vi "Analyzer.TestLauncher.vi"() -> ()   [LabVIEW 2022 SP3, in "Analyzer.lvclass"]
uses:
  Analyzer.lvclass
  Typedefs/Analyzer State--enum.ctl
  <vilib>/JKI/JKI SMO/SMO/Typedefs/SMOState --Enum.ctl
  C:/Program Files (x86)/National Instruments/LabVIEW 2022/vi.lib/JKI/JKI SMO/SMO/SMO.lvclass
  <vilib>/JKI/JKI SMO/SMO/SMO.lvclass/SMO.ctl
  <vilib>/JKI/JKI SMO/SMO/Private/ReftoDVR--SMO.vi
  Analyzer.lvclass/Analyzer.ctl
  <vilib>/JKI/JKI SMO/SMO/SMO.lvclass
panel:
  out "Time":dbl
  out "SMO State":T1
  in  "Embed?":bool=TRUE
  out "UI State":T2
  out "error out":errorcluster
  in  "Stop":bool
  # "SMO.UI_Embedded Test Launcher"
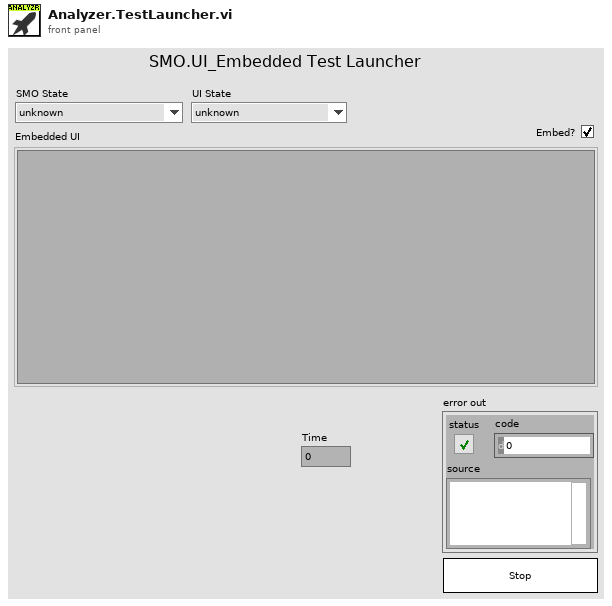
[diagram p1: front panel]
types:
  T1 = typedef "SMO.lvclass/SMOState --Enum.ctl" = enum16{"unknown", "Created", "Started", "Stopped"}
  T2 = typedef "Analyzer.lvclass/Analyzer State--enum.ctl" = enum16{"unknown", "Opened", "Embedded", "Closed"}
  T3 = typedef "SMO.lvclass/Public Events.ctl" = cluster{"Error":refnum<user-event>, "State":refnum<user-event>, "Reserve State":refnum<user-event>}
  T4 = typedef "Analyzer.lvclass/PublicEvents--Cluster.ctl" = cluster{"UI State":refnum<user-event>, "NewEventMessage":refnum<user-event>}
  T5 = cluster{"Event Registration Refnum":refnum<event-registration>}
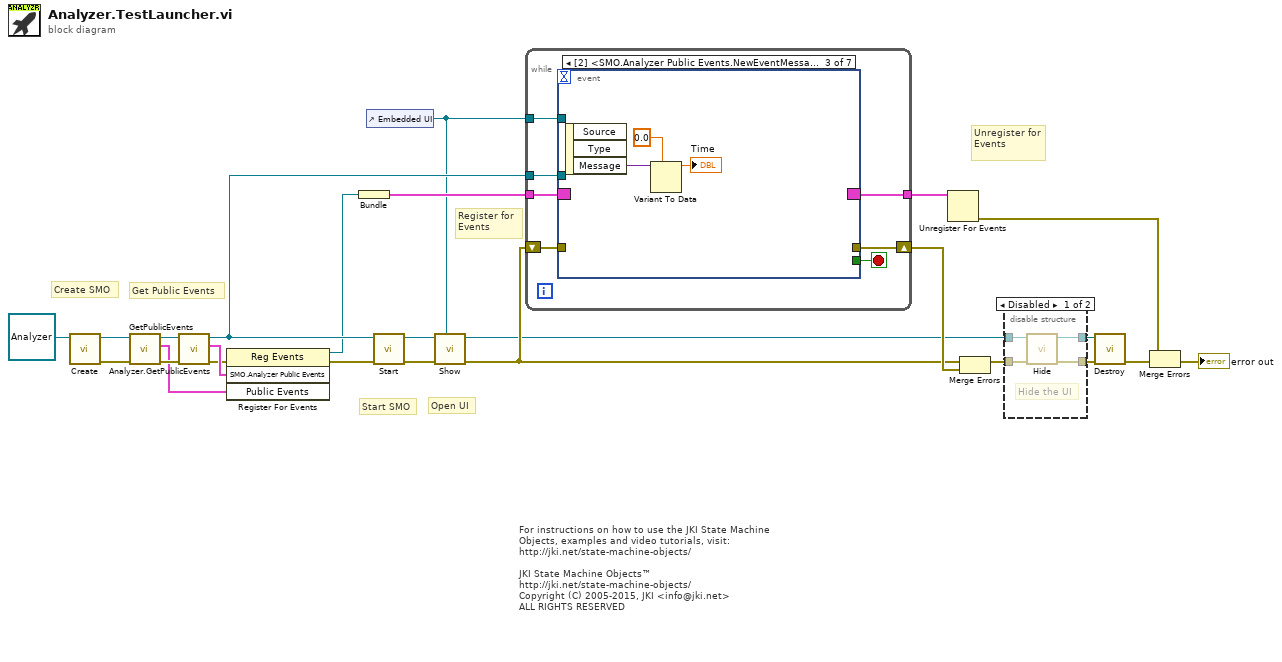
[diagram p0: block diagram]
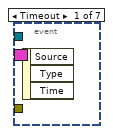
[diagram p3: hidden frame]
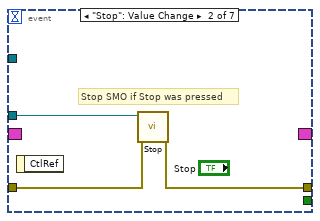
[diagram p4: hidden frame]
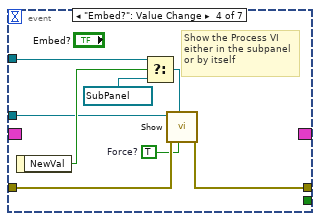
[diagram p5: hidden frame]
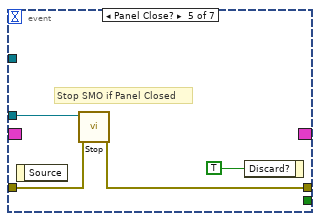
[diagram p6: hidden frame]
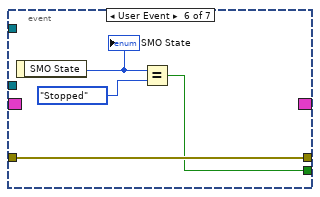
[diagram p7: hidden frame]
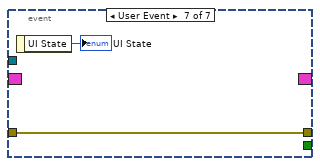
[diagram p8: hidden frame]
diagram:
  # "For instructions on how to use the JKI State Machine Objects, examples and video tutorials, visit:\nhttp://jki.net/state-machine-objects/\n\nJKI State Machine Objects™\nhttp://jki.net/state-machine-objects/\nCopyright (C) 2005-2015, JKI <info@jki.net>\nALL RIGHTS RESERVED"
  # "Get Public Events"
  # "Start SMO"
  # "Create SMO"
  # "Open UI"
  # "Unregister for Events"
  # "Register for Events"
  n1 = call <vilib>:"Create.vi"("SMO"=refnum<class "Analyzer.lvclass"> refnum ("SMO.UI.lvclass")) -> ("error out"=w13:errorcluster, "SMO out"=w11:refnum<class "Analyzer.lvclass">)  [unwired: 8 in, 1 out]
  n2 = call <vilib>:"GetPublicEvents.vi"("error in (no error)"=w13, "SMO"=w11) -> ("error out"=w12:errorcluster, "Public Events"=w9:T3, "SMO out"=w10:refnum<class "Analyzer.lvclass">)  [unwired: 7 in]
  n3 = call "Analyzer.GetPublicEvents.vi"("error in (no error)"=w12, "Analyzer"=w10) -> ("error out"=w15:errorcluster, "SMO.Analyzer Public Events"=w17:T4, "Analyzer out"=w18:refnum<class "Analyzer.lvclass">)  [unwired: 7 in]
  n4 = register-events(error in=w15, w17, w9) -> (reference out=w16:refnum<event-registration>, error out=w14:errorcluster)  [unwired: 1 in]
  n5 = Bundle("Event Registration Refnum"=w16) -> (w24:T5)  [unwired: 1 in]
  n6 = control-ref of="Embedded UI"() -> (w5:refnum<vi>)
  n7 = call <vilib>:"Start.vi"("error in (no error)"=w14, "SMO"=w18) -> ("error out"=w7:errorcluster, "SMO out"=w8:refnum<class "Analyzer.lvclass">)  [unwired: 8 in]
  n8 = call "Show.vi"("Subpanel Ref (empty: open detached)"=w5, "error in (no error)"=w7, "Analyzer"=w8) -> ("error out"=w6:errorcluster, "Analyzer out"=w4:refnum<class "Analyzer.lvclass">)  [unwired: 7 in]
  n9 = while {
    shift-right: [w31] -> w22
    shift-left: w6 -> [w30]
    tunnel: w24 -> [w29]
    tunnel: [w28] -> w25
    tunnel: w18 -> [w27]
    tunnel: w5 -> [w26]
    stop <- w32 stop-if-true
    n10 = event shown="[2] <SMO.Analyzer Public Events.NewEventMessage>: User Event" {
      selector: w29 -> [_ _ _ _ _ _ _]
      dyn-events: [_ _ _ _ _ _ _] -> w28
      timeout: _ -> [_ _ _ _ _ _ _]
      tunnel: [_ _ _ _ _ w51 _] -> w32
      tunnel: w27 -> [_ w33 _ w41 w50 _ _]
      tunnel: [_ w35 _ w46 w49 w52 w56] -> w31
      tunnel: w30 -> [_ w34 _ w40 w48 w52 w56]
      tunnel: w26 -> [_ _ _ w44 _ _ _]
      event Timeout {
        n11 = event-data() -> ()  [unwired: 1 in, 3 out]
      }
      event "Stop": Value Change {
        # "Stop SMO if Stop was pressed"
        n12 = event-data() -> ()  [unwired: 1 in, 1 out]
        n13 = call <vilib>:"Stop.vi"("error in (no error)"=w34, "SMO"=w33) -> ("error out"=w35:errorcluster)  [unwired: 8 in, 1 out]
      }
      event User Event {
        n14 = event-data() -> ("Message"=w38:variant)  [unwired: 1 in, 2 out]
        n15 = Variant To Data(type=0.0, Variant=w38) -> (data=→"Time":dbl)  [unwired: 1 in, 1 out]
      }
      event "Embed?": Value Change {
        w39 = TRUE  # Force?
        # "Show the Process VI\neither in the subpanel\nor by itself"
        n16 = event-data() -> ("NewVal"=w45:bool)  [unwired: 1 in]
        n17 = Select(t=w44, s=w45, f=refnum<vi> refnum) -> (s? t:f=w43:refnum<vi>)
        n18 = call "Show.vi"("Force? (true)"=w39, "Subpanel Ref (empty: open detached)"=w43, "error in (no error)"=w40, "Analyzer"=w41) -> ("error out"=w46:errorcluster)  [unwired: 6 in, 1 out]
      }
      event Panel Close? {
        # "Stop SMO if Panel Closed"
        n19 = event-data() -> ()  [unwired: 1 in, 1 out]
        n20 = call <vilib>:"Stop.vi"("error in (no error)"=w48, "SMO"=w50) -> ("error out"=w49:errorcluster)  [unwired: 8 in, 1 out]
        n21 = event-data("Discard?"=TRUE ("OK")) -> ()  [unwired: 1 in, 1 out]
      }
      event User Event {
        n22 = event-data() -> ("SMO State"=w54:T1)  [unwired: 1 in]
        "SMO State" <- w54
        n23 = Equal?(x=w54, y=SMOState_--Enum."Stopped") -> (x = y?=w51:bool)
      }
      event User Event {
        n24 = event-data() -> ("UI State"=→"UI State":T2)  [unwired: 1 in]
      }
    }
  }
  n25 = Unregister For Events(event registration refnum=w25) -> (error out=w21:errorcluster)  [unwired: 1 in]
  n26 = Merge Errors(w6, w22) -> (w2:errorcluster)
  n27 = disable-structure shown="Disabled" {
    disable-tunnel: w4 -> [w60 w62]
    disable-tunnel: [w59 w62] -> w3
    disable-tunnel: w2 -> [w58 w61]
    disable-tunnel: [w57 w61] -> w1
    frame Disabled {
      # "Hide the UI"
      n28 = call "Hide.vi"("error in (no error)"=w58, "Analyzer"=w60) -> ("error out"=w57:errorcluster, "Analyzer out"=w59:refnum<class "Analyzer.lvclass">)  [unwired: 8 in]
    }
    frame Enabled {
    }
  }
  n29 = call <vilib>:"Destroy.vi"("error in (no error)"=w1, "SMO"=w3) -> ("error out"=w19:errorcluster)  [unwired: 9 in]
  n30 = Merge Errors(w21, w19) -> (→"error out":errorcluster)
